vi "sensor cmd error name.vi"(7 "error_id":u16, 9 "length":i32, 10 "BYTE_ARRAY":string, 11 "device_handle":u32) -> (1 "function return":i32, 2 "BYTE_ARRAY out":string, 3 "device_handle out":u32)   [LabVIEW 2019, in "apdm.lvlib"]
doc: "APDM_EXPORT int apdm_sensor_cmd_error_name(apdm_device_handle_t device_handle, char *BYTE_ARRAY, const int length, uint16_t error_id);"
uses:
  apdm.lvlib
  Lee Lab/CP FES Walking 2018/Code/Working/LabVIEW/apdm.dll
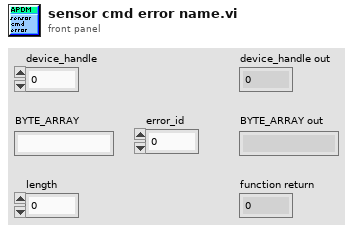
[diagram p1: front panel]
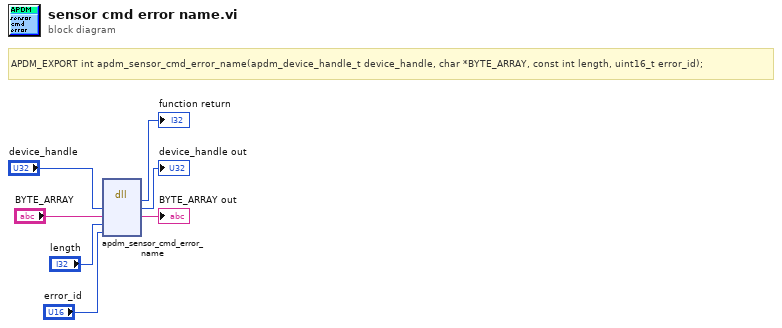
[diagram p0: block diagram]
diagram:
  # "APDM_EXPORT int apdm_sensor_cmd_error_name(apdm_device_handle_t device_handle, char *BYTE_ARRAY, const int length, uint16_t error_id);"
  n1 = dll-call lib="C:/Users/jfalesi/Dropbox/Lee Lab/CP FES Walking 2018/Code/Working/LabVIEW/apdm.*" fn="apdm_sensor_cmd_error_name"("device_handle"="device_handle", "BYTE_ARRAY"="BYTE_ARRAY", "length"="length", "error_id"="error_id") -> (→"function return":i32, "device_handle"=→"device_handle out":u32, "BYTE_ARRAY"=→"BYTE_ARRAY out":string)  [unwired: 5 in, 2 out]
